vi "Read PLC Data.vi"(8 "error in (no error)":errorcluster, 11 "Modbus Master in":refnum<class "Modbus Master.lvclass">) -> (0 "error out":errorcluster, 2 "Ass PLC Data":T2={"Cycle Start Ass"=TRUE, "Bin-1"=TRUE, "Bin-2"=TRUE, "Bin-3"=TRUE, "Bin-4"=TRUE, "Bin-5"=TRUE, "Bin-6"=TRUE, "Bin-7"=TRUE, "Bin-8"=TRUE, "Ass Result OK"=TRUE, "Ass Result NOK"=TRUE, "PLC RUN"=TRUE, "Part Sensor"=TRUE, "Ass Cycle Reset"=TRUE}, 3 "Modbus Master out":refnum<class "Modbus Master.lvclass">, 5 "Torque PLC Data":T1={"Cycle Start Torque"=TRUE, "Bracket-1 Sensor"=TRUE, "Bracket-2 Sensor"=TRUE, "Torquing Result OK"=TRUE, "Torquing Result NOK"=TRUE, "Torquing Cycle Reset"=TRUE, "T-BIN-1"=TRUE, "T-BIN-2"=TRUE, "T-BIN-3"=TRUE, "T-BIN-4"=TRUE, "T-BIN-5"=TRUE, "T-BIN-6"=TRUE})   [LabVIEW 2017]
uses:
  <vilib>/NI/Modbus Library/API/master/Modbus Master.lvclass
  Controls/Ass PLC Data Control.ctl
  Controls/Torque PLC Data Control.ctl
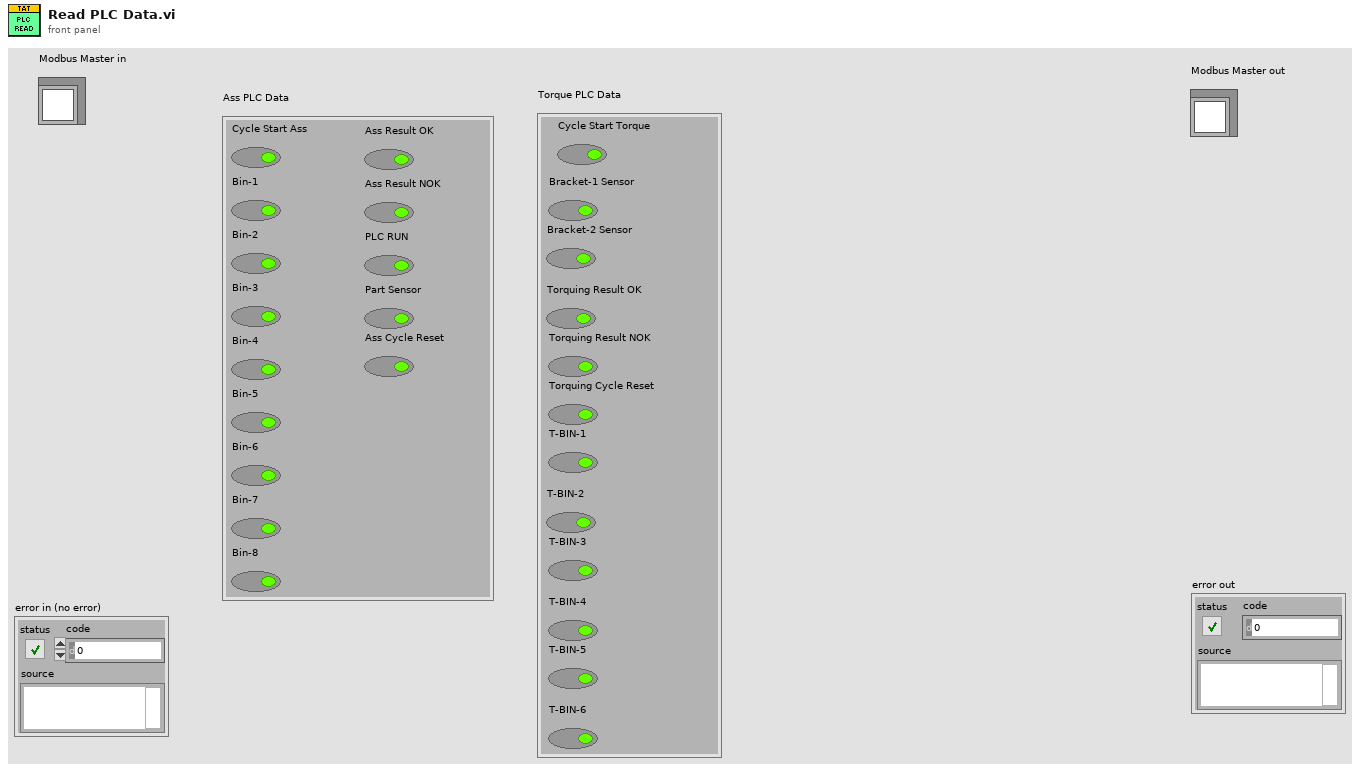
[diagram p1: front panel]
types:
  T1 = typedef "Torque PLC Data Control.ctl" = cluster{"Cycle Start Torque":bool, "Bracket-1 Sensor":bool, "Bracket-2 Sensor":bool, "Torquing Result OK":bool, "Torquing Result NOK":bool, "Torquing Cycle Reset":bool, "T-BIN-1":bool, "T-BIN-2":bool, "T-BIN-3":bool, "T-BIN-4":bool, "T-BIN-5":bool, "T-BIN-6":bool}
  T2 = typedef "Ass PLC Data Control.ctl" = cluster{"Cycle Start Ass":bool, "Bin-1":bool, "Bin-2":bool, "Bin-3":bool, "Bin-4":bool, "Bin-5":bool, "Bin-6":bool, "Bin-7":bool, "Bin-8":bool, "Ass Result OK":bool, "Ass Result NOK":bool, "PLC RUN":bool, "Part Sensor":bool, "Ass Cycle Reset":bool}
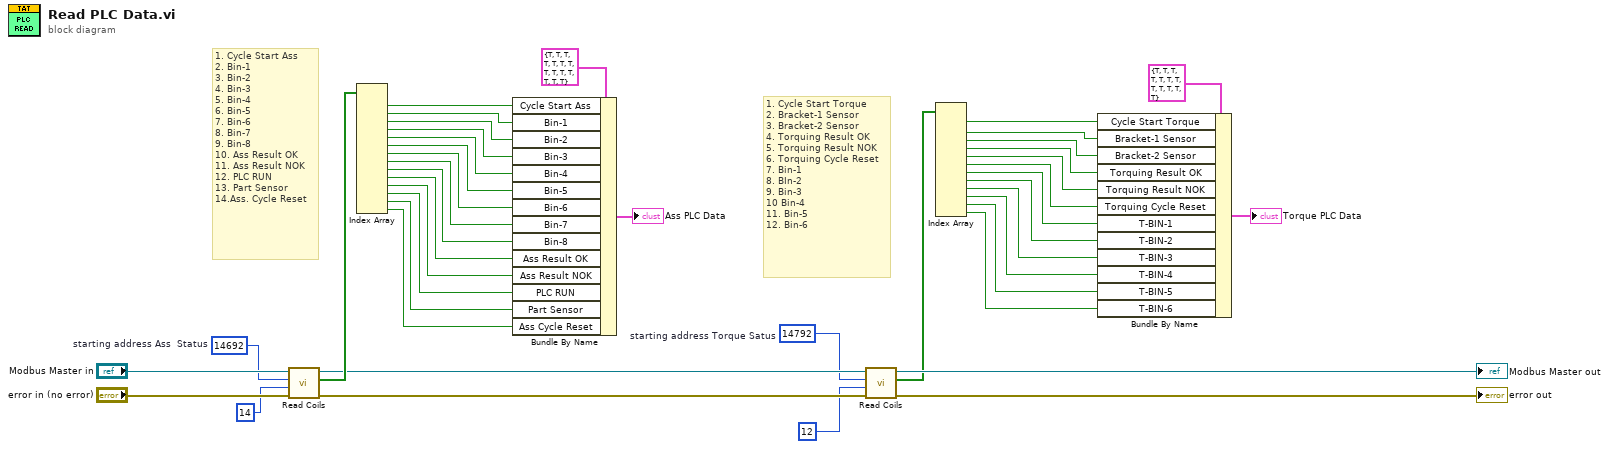
[diagram p0: block diagram]
diagram:
  w17 = u16 14792  # starting address Torque Satus
  w40 = u16 14692  # starting address Ass  Status
  # "1. Cycle Start Torque\n2. Bracket-1 Sensor\n3. Bracket-2 Sensor\n4. Torquing Result OK\n5. Torquing Result NOK\n6. Torquing Cycle Reset\n7. Bin-1\n8. BIn-2\n9. Bin-3\n10 Bin-4\n11. Bin-5\n12. Bin-6"
  # "1. Cycle Start Ass\n2. Bin-1\n3. Bin-2\n4. Bin-3\n5. Bin-4\n6. Bin-5\n7. Bin-6\n8. Bin-7\n9. Bin-8\n10. Ass Result OK\n11. Ass Result NOK\n12. PLC RUN\n13. Part Sensor\n14.Ass. Cycle Reset"
  n1 = call-dynamic "Read Coils.vi"("error in"="error in (no error)", "number of inputs"=u16 14, "starting address"=w40, "Modbus master in"="Modbus Master in") -> ("error out"=w20:errorcluster, "coils"=w37:bool[], "Modbus master out"=w21:refnum<class "Modbus Master.lvclass">)  [unwired: 5 in]
  n2 = Index Array(array=w37) -> (element #1=w36:bool, element #2=w35:bool, element #3=w34:bool, element #4=w33:bool, element #5=w32:bool, element #6=w31:bool, element #7=w30:bool, element #8=w29:bool, element #9=w28:bool, element #10=w27:bool, element #11=w26:bool, element #12=w25:bool, element #13=w24:bool, element #14=w22:bool)  [unwired: 14 in]
  n3 = Bundle By Name(cluster=T2 {"Cycle Start Ass"=TRUE, "Bin-1"=TRUE, "Bin-2"=TRUE, "Bin-3"=TRUE, "Bin-4"=TRUE, "Bin-5"=TRUE, "Bin-6"=TRUE, "Bin-7"=TRUE, "Bin-8"=TRUE, "Ass Result OK"=TRUE, "Ass Result NOK"=TRUE, "PLC RUN"=TRUE, "Part Sensor"=TRUE, "Ass Cycle Reset"=TRUE}, "Cycle Start Ass"=w36, "Bin-1"=w35, "Bin-2"=w34, "Bin-3"=w33, "Bin-4"=w32, "Bin-5"=w31, "Bin-6"=w30, "Bin-7"=w29, "Bin-8"=w28, "Ass Result OK"=w27, "Ass Result NOK"=w26, "PLC RUN"=w25, "Part Sensor"=w24, "Ass Cycle Reset"=w22) -> (→"Ass PLC Data":T2)
  n4 = call-dynamic "Read Coils.vi"("error in"=w20, "number of inputs"=u16 12, "starting address"=w17, "Modbus master in"=w21) -> ("error out"=→"error out":errorcluster, "coils"=w15:bool[], "Modbus master out"=→"Modbus Master out":refnum<class "Modbus Master.lvclass">)  [unwired: 5 in]
  n5 = Index Array(array=w15) -> (element #1=w13:bool, element #2=w12:bool, element #3=w11:bool, element #4=w10:bool, element #5=w9:bool, element #6=w8:bool, element #7=w6:bool, element #8=w5:bool, element #9=w4:bool, element #10=w3:bool, element #11=w2:bool, element #12=w1:bool)  [unwired: 12 in]
  n6 = Bundle By Name(cluster=T1 {"Cycle Start Torque"=TRUE, "Bracket-1 Sensor"=TRUE, "Bracket-2 Sensor"=TRUE, "Torquing Result OK"=TRUE, "Torquing Result NOK"=TRUE, "Torquing Cycle Reset"=TRUE, "T-BIN-1"=TRUE, "T-BIN-2"=TRUE, "T-BIN-3"=TRUE, "T-BIN-4"=TRUE, "T-BIN-5"=TRUE, "T-BIN-6"=TRUE}, "Cycle Start Torque"=w13, "Bracket-1 Sensor"=w12, "Bracket-2 Sensor"=w11, "Torquing Result OK"=w10, "Torquing Result NOK"=w9, "Torquing Cycle Reset"=w8, "T-BIN-1"=w6, "T-BIN-2"=w5, "T-BIN-3"=w4, "T-BIN-4"=w3, "T-BIN-5"=w2, "T-BIN-6"=w1) -> (→"Torque PLC Data":T1)
